vi "Read File.vi"(8 "error in (no error)":errorcluster, 11 "Refnum in":T1) -> (0 "error out":errorcluster, 2 "value":string, 3 "value 2":i32)   [LabVIEW 2020]
uses:
  <vilib>/Utility/config.llb/Config Data RefNum.ctl
  <vilib>/Utility/config.llb/Read Key (I32).vi
  <vilib>/Utility/config.llb/Read Key (String).vi
  <vilib>/Utility/config.llb/NI_LVConfig.lvlib
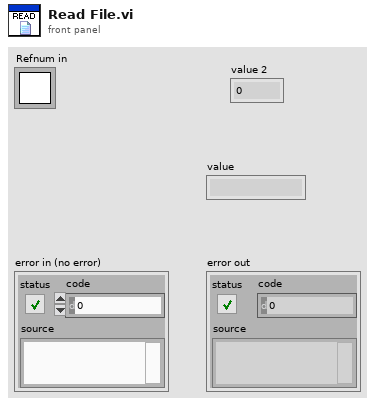
[diagram p1: front panel]
types:
  T1 = typedef "NI_LVConfig.lvlib/Config Data RefNum.ctl" = refnum<k1>
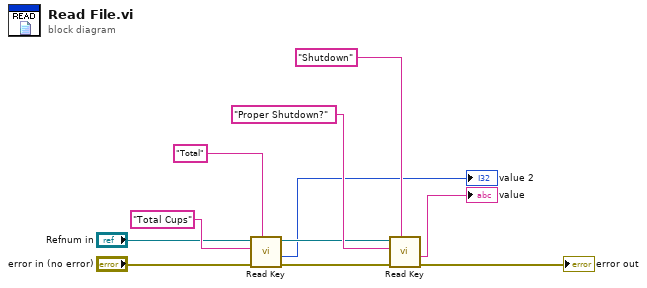
[diagram p0: block diagram]
diagram:
  n1 = call-poly <vilib>:"Read Key.vi"("section"="Total", "error in (no error)"="error in (no error)", "key"="Total Cups", "refnum"="Refnum in") -> ("error out"=w6:errorcluster, "value"=→"value 2":i32, "refnum out"=w8:T1)  [unwired: 4 in, 1 out]
  n2 = call-poly <vilib>:"Read Key.vi"("section"="Shutdown" ("String"), "error in (no error)"=w6, "key"="Proper Shutdown?", "refnum"=w8) -> ("error out"=→"error out":errorcluster, "value"=→"value":string)  [unwired: 4 in, 2 out]
